vi "Write Sense_Point.vi"(8 "error in":errorcluster, 10 "Sense Point":T1, 11 "6700C in":refnum<class "6700C.lvclass">) -> (0 "error out":errorcluster, 3 "6700C out":refnum<class "6700C.lvclass">)   [LabVIEW 2019, in "6700C.lvlib" / "6700C.lvclass"]
uses:
  Library/6700C.lvclass
  C:/Users/Public/Documents/Development/builds/Engine/Monitored Actor.lvlibp/Monitored Actor/Monitored Actor/Monitored Actor.lvclass
  builds/Instruments/PowerSupply.lvlibp/Custom Controls/Sense Point.ctl
  builds/Engine/Monitored Actor.lvlibp/Monitored Actor/Monitored Actor/Read Actor Label.vi
  builds/Instruments/PowerSupply.lvlibp/Library/PowerSupply.lvclass
  <vilib>/ErrorRing/Error Ring.xnode
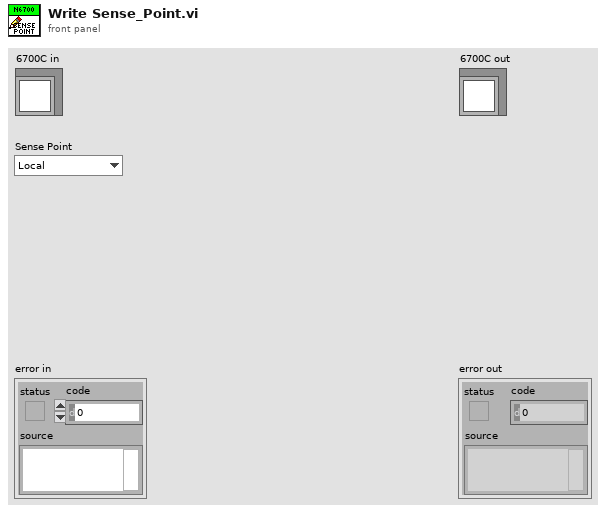
[diagram p1: front panel]
types:
  T1 = typedef "PowerSupply.lvlibp/PowerSupply.lvclass/Sense Point.ctl" = enum16{"Local", "Remote"}
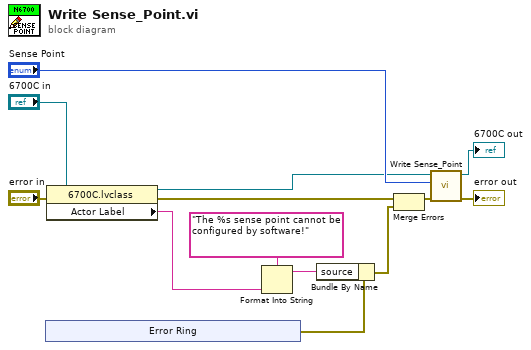
[diagram p0: block diagram]
diagram:
  n1 = xnode "Error Ring"() -> ("error out"=w10:errorcluster)
  n2 = property class="6700C.lvclass"(reference="6700C in", error in="error in") -> (reference out=w3:refnum<class "6700C.lvclass">, error out=w2:errorcluster, "Actor Label"=w1:string)
  n3 = Format Into String(format string="The %s sense point cannot be configured by software!", w1) -> (resulting string=w9:string)  [unwired: 2 in, 1 out]
  n4 = Bundle By Name(cluster=w10, "source"=w9) -> (w6:errorcluster)
  n5 = Merge Errors(w2, w6) -> (w7:errorcluster)
  n6 = call-parent "Write Sense_Point.vi"("error in"=w7, "Sense Point"="Sense Point", "PowerSupply in"=w3) -> ("error out"=→"error out":errorcluster, "PowerSupply out"=→"6700C out":refnum<class "6700C.lvclass">)  [unwired: 7 in]
